vi "CMC_Simple_AAP.vi"() -> ()   [LabVIEW 2013]
panel:
  out "Average Value":dbl format="%#_3g"
  out "Waveform Graph":dynamicdata(graph)
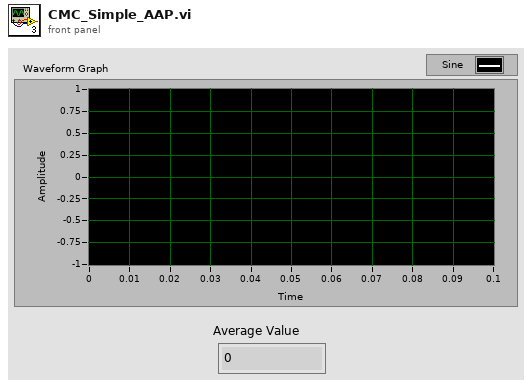
[diagram p1: front panel]
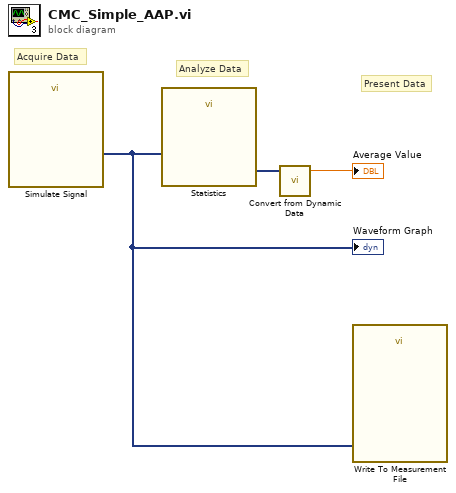
[diagram p0: block diagram]
diagram:
  # "Present Data"
  # "Analyze Data"
  # "Acquire Data"
  n1 = call "Simulate Signal"() -> ("Sine"=w1:dynamicdata)  [unwired: 14 in, 1 out]
  "Waveform Graph" <- w1
  n2 = call "Statistics"("Signals"=w1) -> ("Arithmetic Mean"=w2:dynamicdata)  [unwired: 25 in, 1 out]
  n3 = call "Convert from Dynamic Data"("Dynamic Data Type"=w2) -> ("Scalar"=→"Average Value":dbl)  [unwired: 3 in]
  n4 = call "Write To Measurement File"("Signals"=w1) -> ()  [unwired: 16 in, 3 out]
